vi "niRFUtil FTW Generate AAF FIR Filter.vi"(0 "Input Sample Rate (Hz)":dbl=1.0 format="%^.3e", 5 "Desired Sample Rate (Hz)":dbl=1.0 format="%^.3e") -> (4 "Anti Alias Filter":T1 {"y" min=0 max=127 format="%.2f"; "dx" format="%^.2e"; "x0" format="%^.2e"})   [LabVIEW 2015, in "niRFUtil.lvlib"]
uses:
  niRFUtil.lvlib
  Includes/niRFUtil INC Real Waveform.ctl
  Includes/niRFUtil INC Real Array.ctl
  <vilib>/Analysis/3filter.llb/Filter Passband Type.ctl
  <vilib>/Analysis/4window.llb/windowTd.ctl
  <vilib>/Analysis/NI_AALBase.lvlib
  <vilib>/Analysis/NI_AALPro.lvlib
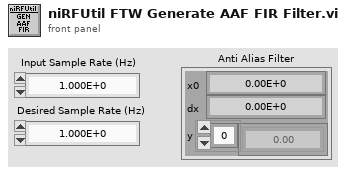
[diagram p1: front panel]
types:
  T1 = typedef "niRFUtil.lvlib/niRFUtil INC Real Waveform.ctl" = cluster{"x0":dbl, "dx":dbl, "y":T2}
  T2 = typedef "niRFUtil.lvlib/niRFUtil INC Real Array.ctl" = sgl[]
  T3 = typedef "NI_AALBase.lvlib/Filter Passband Type.ctl" = enum32{"Lowpass", "Highpass", "Bandpass", "Bandstop"}
  T4 = typedef "NI_AALPro.lvlib/windowTd.ctl" = u32
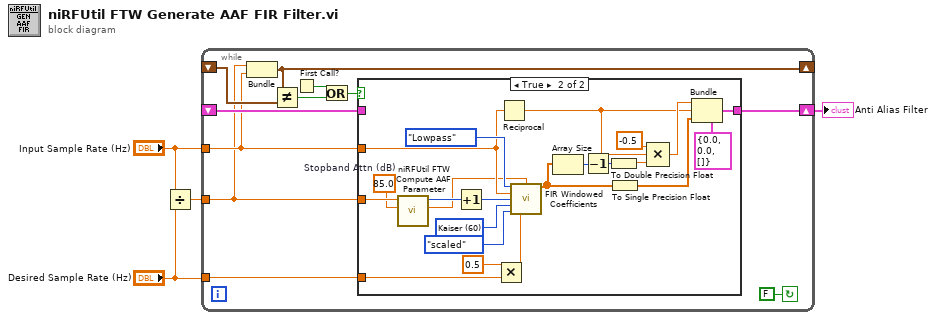
[diagram p0: block diagram]
diagram:
  n1 = Divide(x="Input Sample Rate (Hz)", y="Desired Sample Rate (Hz)") -> (x/y=w4:dbl)
  n2 = while {
    tunnel: w4 -> [w8]
    tunnel: "Input Sample Rate (Hz)" -> [w9]
    tunnel: "Desired Sample Rate (Hz)" -> [w14]
    shift-right: [w15] -> w1
    shift-left: _ -> [w10]
    shift-right: [w13] -> _
    shift-left: _ -> [w12]
    stop <- FALSE continue-if-true
    n3 = Bundle(w8, "Input Sample Rate (Hz)"=w9) -> (w13:cluster{dbl, "Input Sample Rate (Hz)":dbl})  [unwired: 1 in]
    n4 = Not Equal?(x=w13, y=w12) -> (x != y?=w6:bool)
    n5 = First Call?() -> (First Call?: T/F=w7:bool)
    n6 = Or(x=w7, y=w6) -> (x .or. y?=w5:bool)
    n7 = case shown="True" w5 {
      tunnel: [w16 w27] -> w15
      tunnel: w9 -> [_ w23]
      tunnel: w14 -> [_ w20]
      tunnel: w10 -> [w16 _]
      tunnel: w8 -> [_ w21]
      frame False {
      }
      frame True {
        w17 = 85.0  # Stopband Attn (dB)
        w29 = T4 60 items=["Rectangle"=0, "Hanning"=1, "Hamming"=2, "Blackman-Harris"=3, "Exact Blackman"=4, "Blackman"=5, "Flat Top"=6, "4 Term B-Harris "=7, "7 Term B-Harris"=8, "Low Sidelobe"=9, "Blackman Nuttall"=11, "Triangle"=30, "Bartlett-Hanning"=31, "Bohman"=32, "Parzen"=33, "Welch"=34, "Kaiser"=60, "Dolph-Chebyshev"=61, "Gaussian"=62] ("window")
        n8 = call "niRFUtil FTW Compute AAF Parameter.vi"("Stopband Attenuation (dB)"=w17, "Decimation Rate"=w21) -> ("Kaiser Beta"=w18:dbl, "AAF Order"=w19:i32)  [unwired: 8 in]
        n9 = Increment(x=w19) -> (x+1=w22:i32)
        n10 = Multiply(x=0.5 ("y"), y=w20) -> (x*y=w32:dbl)
        n11 = Reciprocal(x=w23) -> (1/x=w25:dbl)
        n12 = call <vilib>:"FIR Windowed Coefficients.vi"("filter type"=Filter_Passband_Type."Lowpass", "window parameter"=w18, "sampling freq: fs"=w23, "taps"=w22, "window"=w29, "option"=enum32{"not scaled", "scaled"}."scaled", "low cutoff freq: fl"=w32) -> ("FIR Windowed Coefficients"=w33:dbl[])  [unwired: 7 in, 1 out]
        n13 = Array Size(array=w33) -> (size(s)=w34:i32)
        n14 = Decrement(x=w34) -> (x-1=w35:i32)
        n15 = To Double Precision Float(number=w35) -> (double precision float=w36:dbl)
        n16 = To Single Precision Float(number=w33) -> (single precision float=w24:sgl[])
        n17 = Compound Arithmetic op=MULTIPLY(-0.5 ("value"), w25, w36) -> (w38:dbl)
        n18 = Bundle(cluster=T1 {"x0"=0.0, "dx"=0.0, "y"=[]} ("Real Waveform"), "x0"=w38, "dx"=w25, "y"=w24) -> (w27:T1)
      }
    }
  }
  "Anti Alias Filter" <- w1
